vi "Test Sequencer.vi"() -> ()   [LabVIEW 2021]
uses:
  System/bt_System.lvclass
  <vilib>/TSA/Event Log/Event_TextLog/Event_TextLog.lvclass/Event_TextLog.ctl
  <vilib>/numeric/Random Number (Range) DBL.vi
  <vilib>/TSA/Abstract Data Classes/Abs_Types/Boolean/Simple Read.vi
  <vilib>/TSA/Abstract Data Classes/Abs_Types/Double Float/Static Write.vi
  <vilib>/TSA/Abstract Data Classes/Abs_Types/Waveform/Static Write.vi
  <vilib>/TSA/Abstract Data Classes/Abs_Types/Boolean/Static Write.vi
  <vilib>/TSA/Abstract Data Classes/Abs_Types/Waveform/Abs_Waveform.lvclass
  <vilib>/TSA/Abstract Data Classes/Abs_Types/Boolean/Abs_Boolean.lvclass
  <vilib>/TSA/Abstract Data Classes/Abs_Types/Double Float/Abs_Double Float.lvclass
  <vilib>/TSA/Event Log/Event_TextLog/Event_TextLog.lvclass
  Blackboard/Blackboard.lvclass
  Support/Test Sequencer Support.lvlib
  <vilib>/measure/NI_MABase.lvlib
panel:
  out "Fail Indicator":bool
  out "Pass Indicator":bool
  out "Reading":dbl format="%.2g"
  in  "Amplitude":dbl(slide)=4.74025974025974 scale=0.0..10.0
  in  "Frequency (Hz)":dbl(slide)=10.150641893704565 scale=0.1..100.0
  in  "Voltage":dbl(slide)=5.3896103896103895 scale=0.0..10.0
  out "Waveform Graph":waveform(dbl)(graph)
  in  "Start Test":bool
  out "Log Message":string
  in  "Stop":bool
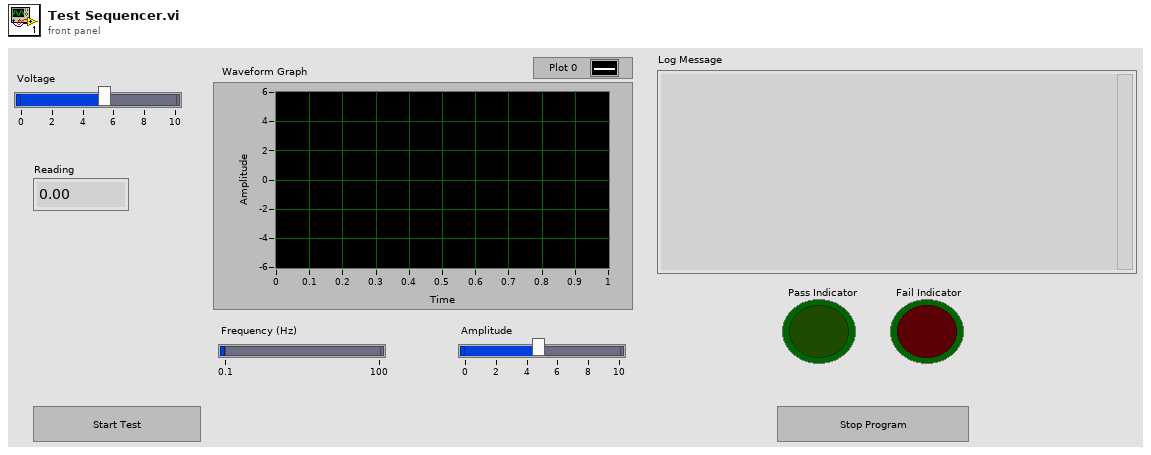
[diagram p1: front panel]
types:
  T1 = typedef "Test Sequencer Support.lvlib/IO Type.ctl" = cluster{"Log":refnum<class "Event_TextLog.lvclass">, "Blackboard":refnum<class "Blackboard.lvclass">, "Start Test":refnum<class "Abs_Boolean.lvclass">, "Measurements":cluster{"Waveform":refnum<class "Abs_Waveform.lvclass">, "Voltage":refnum<class "Abs_Double Float.lvclass">, "Measured Frequency":refnum<class "Abs_Double Float.lvclass">, "Measured Amplitude":refnum<class "Abs_Double Float.lvclass">}, "Pass Status":refnum<class "Abs_Boolean.lvclass">, "Fail Status":refnum<class "Abs_Boolean.lvclass">}
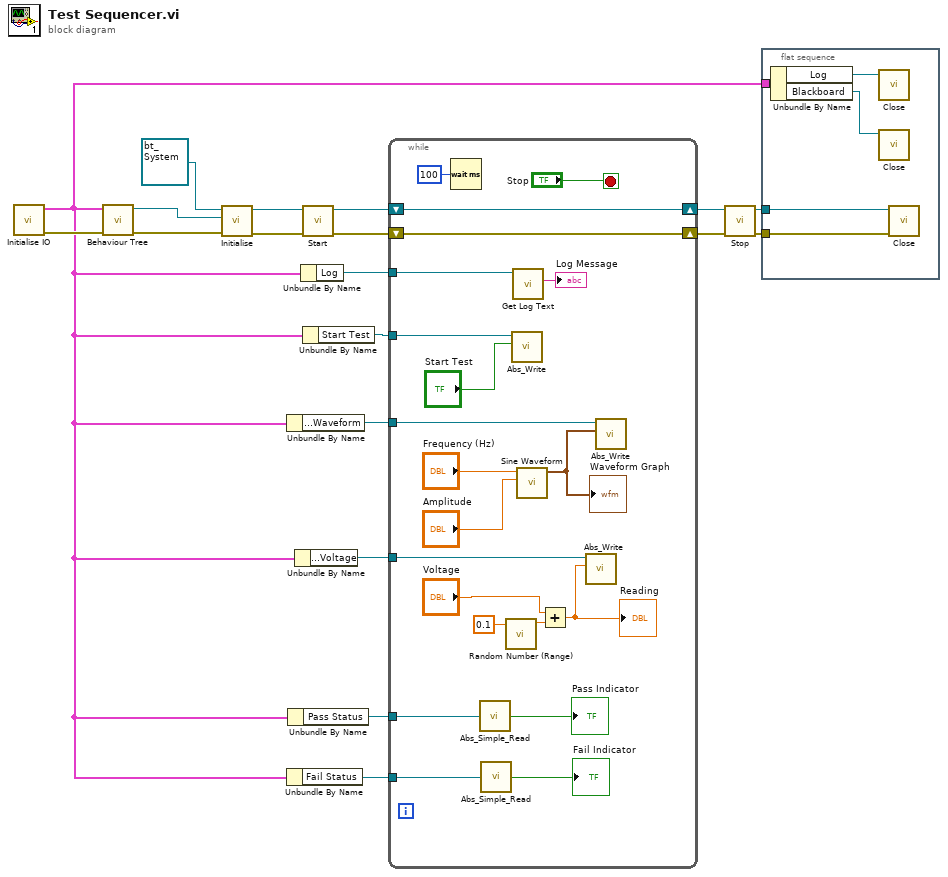
[diagram p0: block diagram]
diagram:
  n1 = call "Initialise IO.vi"() -> ("error out"=w8:errorcluster, "IO"=w1:T1)  [unwired: 10 in]
  n2 = call "Behaviour Tree.vi"("IO"=w1) -> ("bt_Node out"=w9:refnum<class "bt_Node.lvclass">)  [unwired: 10 in]
  n3 = call "Initialise.vi"("error in (no error)"=w8, "Behaviour Tree"=w9, "bt_System in"=refnum<class "bt_System.lvclass"> refnum) -> ("error out"=w16:errorcluster, "bt_System out"=w17:refnum<class "bt_System.lvclass">)  [unwired: 7 in]
  n4 = Unbundle By Name(w1) -> ("Measurements.Waveform"=w5:refnum<class "Abs_Waveform.lvclass">)
  n5 = Unbundle By Name(w1) -> ("Fail Status"=w2:refnum<class "Abs_Boolean.lvclass">)
  n6 = Unbundle By Name(w1) -> ("Pass Status"=w3:refnum<class "Abs_Boolean.lvclass">)
  n7 = Unbundle By Name(w1) -> ("Measurements.Voltage"=w4:refnum<class "Abs_Double Float.lvclass">)
  n8 = Unbundle By Name(w1) -> ("Log"=w7:refnum<class "Event_TextLog.lvclass">)
  n9 = call "Start.vi"("error in (no error)"=w16, "bt_System in"=w17) -> ("error out"=w14:errorcluster, "bt_System out"=w15:refnum<class "bt_System.lvclass">)  [unwired: 8 in]
  n10 = Unbundle By Name(w1) -> ("Start Test"=w6:refnum<class "Abs_Boolean.lvclass">)
  n11 = while {
    shift-right: [w39] -> w13
    shift-left: w15 -> [w39]
    shift-right: [w38] -> w12
    shift-left: w14 -> [w38]
    tunnel: w7 -> [w34]
    tunnel: w6 -> [w33]
    tunnel: w5 -> [w28]
    tunnel: w4 -> [w27]
    tunnel: w3 -> [w22]
    tunnel: w2 -> [w20]
    stop <- "Stop" stop-if-true
    n12 = Wait (ms)(milliseconds to wait=u32 100) -> ()  [unwired: 1 out]
    n13 = call-poly <vilib>:"Abs_Simple_Read.vi"("Boolean in"=w22) -> ("Boolean"=→"Pass Indicator":bool)  [unwired: 4 in]
    n14 = call-poly <vilib>:"Abs_Simple_Read.vi"("Boolean in"=w20) -> ("Boolean"=→"Fail Indicator":bool)  [unwired: 4 in]
    n15 = call-poly <vilib>:"Random Number (Range).vi"("upper bound (100)"=0.1) -> ("number"=w25:dbl)  [unwired: 10 in]
    n16 = call-poly <vilib>:"Abs_Write.vi"("Boolean"="Start Test", "Abs_Boolean in"=w33) -> ()  [unwired: 8 in, 2 out]
    n17 = call <vilib>:"Get Log Text.vi"("Event_TextLog in"=w34) -> ("Log Message"=→"Log Message":string)  [unwired: 8 in, 2 out]
    n18 = call <vilib>:"Sine Waveform.vi"("amplitude"="Amplitude", "frequency"="Frequency (Hz)") -> ("signal out"=w29:waveform(dbl))  [unwired: 8 in, 1 out]
    "Waveform Graph" <- w29
    n19 = Add(x="Voltage", y=w25) -> (x+y=w23:dbl)
    "Reading" <- w23
    n20 = call-poly <vilib>:"Abs_Write.vi"("Value"=w23, "Abs_Double Float in"=w27) -> ()  [unwired: 8 in, 2 out]
    n21 = call-poly <vilib>:"Abs_Write.vi"("Waveform"=w29, "Abs_Waveform in"=w28) -> ()  [unwired: 8 in, 2 out]
  }
  n22 = call "Stop.vi"("error in (no error)"=w12, "bt_System in"=w13) -> ("error out"=w10:errorcluster, "bt_System out"=w11:refnum<class "bt_System.lvclass">)  [unwired: 8 in]
  n23 = flat-sequence {
    tunnel: w11 -> [w44]
    tunnel: w10 -> [w43]
    tunnel: w1 -> [w42]
    frame #0 {
      n24 = Unbundle By Name(w42) -> ("Log"=w41:refnum<class "Event_TextLog.lvclass">, "Blackboard"=w40:refnum<class "Blackboard.lvclass">)
      n25 = call-dynamic "Close.vi"("Event_TextLog in"=w41) -> ()  [unwired: 9 in, 2 out]
      n26 = call-dynamic "Close.vi"("bt_Blackboard in"=w40) -> ()  [unwired: 9 in, 2 out]
      n27 = call-dynamic "Close.vi"("error in (no error)"=w43, "bt_System in"=w44) -> ()  [unwired: 8 in, 2 out]
    }
  }
